vi "Moving-Average.vi"(1 "Average number":i32=8, 2 "X":dbl[](array[numeric])) -> (0 "Filtered X":dbl[](array[numeric]))   [LabVIEW 2013]
uses:
  <vilib>/Analysis/3filter.llb/FIR Filter (DBL).vi
  <vilib>/Analysis/NI_AALBase.lvlib
panel:
  out "Result":cluster{"X":dbl[]}[](graph)
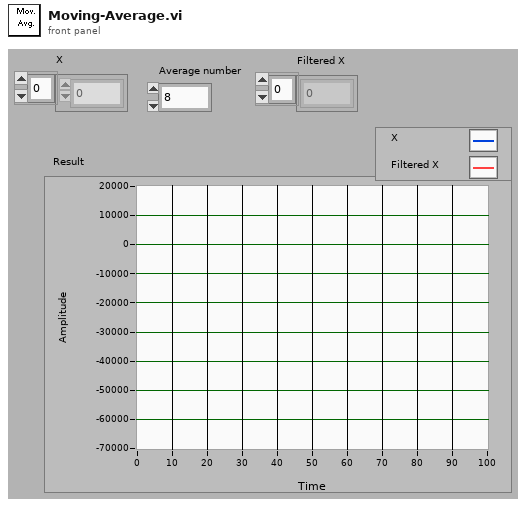
[diagram p1: front panel]
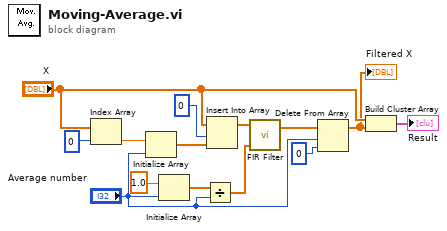
[diagram p0: block diagram]
diagram:
  n1 = Index Array(array="X", index=0) -> (element=w9:dbl)
  n2 = Initialize Array(w9, "Average number") -> (w8:dbl[])
  n3 = Initialize Array(1.0 ("element"), "Average number") -> (w12:dbl[])
  n4 = Divide(x=w12, y="Average number") -> (x/y=w13:dbl[])
  n5 = Insert Into Array(array="X", index=0, new element=w8) -> (w7:dbl[])
  n6 = call-poly <vilib>:"FIR Filter.vi"("FIR Coefficients"=w13, "X"=w7) -> ("Filtered X"=w6:dbl[])  [unwired: 1 in, 2 out]
  n7 = Delete From Array(array=w6, length="Average number", index=0) -> (array with subset deleted=w1:dbl[])  [unwired: 1 out]
  "Filtered X" <- w1
  n8 = Build Cluster Array("X", w1) -> (→"Result":cluster{"Filtered X":dbl[]}[])
